vi "testing_delay_sweep_multifold_4ch.vi"() -> ()   [LabVIEW 2015, in "Tausand AB1000.lvlib"]
uses:
  <instrlib>/Tausand AB1000/Public/Controls/counters4ch.ctl
  <instrlib>/Tausand AB1000/Public/Controls/channelRing.ctl
  <instrlib>/Tausand AB1000/Public/Controls/configMultipleCoincRing.ctl
  <instrlib>/Tausand AB1000/Public/Controls/deviceTypeRing.ctl
  <instrlib>/Tausand AB1000/Tausand AB1000.lvlib
panel:
  out "device type":T1 items=["any"=0, "AB1002"=1002, "AB1004"=1004, "AB1502"=1502, "AB1504"=1504, "AB2002"=2002, "AB2004"=2004, "AB2502"=2502, "AB2504"=2504]
  out "multifold case":T2[](array[typedef])=[240, 224, 208, 176, 112] items=["ABC"=224, "ABD"=208, "ABE"=200, "ABF"=196, "ABG"=194, "ABH"=193, "ACD"=176, "ACE"=168, "ACF"=164, "ACG"=162, "ACH"=161, "ADE"=152, "ADF"=148, "ADG"=146, "ADH"=145, "AEF"=140, "AEG"=138, "AEH"=137, "AFG"=134, "AFH"=133, "AGH"=131, "BCD"=112, "BCE"=104, "BCF"=100, "BCG"=98, "BCH"=97, "BDE"=88, "BDF"=84, "BDG"=82, "BDH"=81, "BEF"=76, "BEG"=74, "BEH"=73, "BFG"=70, "BFH"=69, "BGH"=67, "CDE"=56, "CDF"=52, "CDG"=50, "CDH"=49, "CEF"=44, "CEG"=42, "CEH"=41, "CFG"=38, "CFH"=37, "CGH"=35, "DEF"=28, "DEG"=26, "DEH"=25, "DFG"=22, "DFH"=21, "DGH"=19, "EFG"=14, "EFH"=13, "EGH"=11, "FGH"=7, "ABCD"=240, "ABCE"=232, "ABCF"=228, "ABCG"=226, "ABCH"=225, "ABDE"=216, "ABDF"=212, "ABDG"=210, "ABDH"=209, "ABEF"=204, "ABEG"=202, "ABEH"=201, "ABFG"=198, "ABFH"=197, "ABGH"=195, "ACDE"=184, "ACDF"=180, "ACDG"=178, "ACDH"=177, "ACEF"=172, "ACEG"=170, "ACEH"=169, "ACFG"=166, "ACFH"=165, "ACGH"=163, "ADEF"=156, "ADEG"=154, "ADEH"=153, "ADFG"=150, "ADFH"=149, "ADGH"=147, "AEFG"=142, "AEFH"=141, "AEGH"=139, "AFGH"=135, "BCDE"=120, "BCDF"=116, "BCDG"=114, "BCDH"=113, "BCEF"=108, "BCEG"=106, "BCEH"=105, "BCFG"=102, "BCFH"=101, "BCGH"=99, "BDEF"=92, "BDEG"=90, "BDEH"=89, "BDFG"=86, "BDFH"=85, "BDGH"=83, "BEFG"=78, "BEFH"=77, "BEGH"=75, "BFGH"=71, "CDEF"=60, "CDEG"=58, "CDEH"=57, "CDFG"=54, "CDFH"=53, "CDGH"=51, "CEFG"=46, "CEFH"=45, "CEGH"=43, "CFGH"=39, "DEFG"=30, "DEFH"=29, "DEGH"=27, "DFGH"=23, "EFGH"=15]
  out "tausand data":u32[][](array[numeric])
  out "current multifold":T2=224 caption="Current multifold" items=["ABC"=224, "ABD"=208, "ABE"=200, "ABF"=196, "ABG"=194, "ABH"=193, "ACD"=176, "ACE"=168, "ACF"=164, "ACG"=162, "ACH"=161, "ADE"=152, "ADF"=148, "ADG"=146, "ADH"=145, "AEF"=140, "AEG"=138, "AEH"=137, "AFG"=134, "AFH"=133, "AGH"=131, "BCD"=112, "BCE"=104, "BCF"=100, "BCG"=98, "BCH"=97, "BDE"=88, "BDF"=84, "BDG"=82, "BDH"=81, "BEF"=76, "BEG"=74, "BEH"=73, "BFG"=70, "BFH"=69, "BGH"=67, "CDE"=56, "CDF"=52, "CDG"=50, "CDH"=49, "CEF"=44, "CEG"=42, "CEH"=41, "CFG"=38, "CFH"=37, "CGH"=35, "DEF"=28, "DEG"=26, "DEH"=25, "DFG"=22, "DFH"=21, "DGH"=19, "EFG"=14, "EFH"=13, "EGH"=11, "FGH"=7, "ABCD"=240, "ABCE"=232, "ABCF"=228, "ABCG"=226, "ABCH"=225, "ABDE"=216, "ABDF"=212, "ABDG"=210, "ABDH"=209, "ABEF"=204, "ABEG"=202, "ABEH"=201, "ABFG"=198, "ABFH"=197, "ABGH"=195, "ACDE"=184, "ACDF"=180, "ACDG"=178, "ACDH"=177, "ACEF"=172, "ACEG"=170, "ACEH"=169, "ACFG"=166, "ACFH"=165, "ACGH"=163, "ADEF"=156, "ADEG"=154, "ADEH"=153, "ADFG"=150, "ADFH"=149, "ADGH"=147, "AEFG"=142, "AEFH"=141, "AEGH"=139, "AFGH"=135, "BCDE"=120, "BCDF"=116, "BCDG"=114, "BCDH"=113, "BCEF"=108, "BCEG"=106, "BCEH"=105, "BCFG"=102, "BCFH"=101, "BCGH"=99, "BDEF"=92, "BDEG"=90, "BDEH"=89, "BDFG"=86, "BDFH"=85, "BDGH"=83, "BEFG"=78, "BEFH"=77, "BEGH"=75, "BFGH"=71, "CDEF"=60, "CDEG"=58, "CDEH"=57, "CDFG"=54, "CDFH"=53, "CDGH"=51, "CEFG"=46, "CEFH"=45, "CEGH"=43, "CFGH"=39, "DEFG"=30, "DEFH"=29, "DEGH"=27, "DFGH"=23, "EFGH"=15]
  in  "delayed channel":T3=1 items=["none", "A", "B", "C", "D", "E", "F", "G", "H"]
  in  "cw (ns)":u32=2
  out "i case":i32
  out "total cases":i32
  in  "Stop Button":bool
  out "coinc Chart":T4(graph)
  out "current values":T5
  in  "sampling (ms)":u32=1000
  out "i delay":i32
  out "delay array":u32[](array[numeric])
  in  "step delay":u32=2
  in  "max delay":u32=10
  in  "min delay":u32
  out "current delay (ns)":u32
  in  "VISA resource name":refnum<visa-resource-name>
  # "delayA"
  # "delayB"
  # "delayC"
  # "delayD"
  # "c.win."
  # "case"
  # "out of"
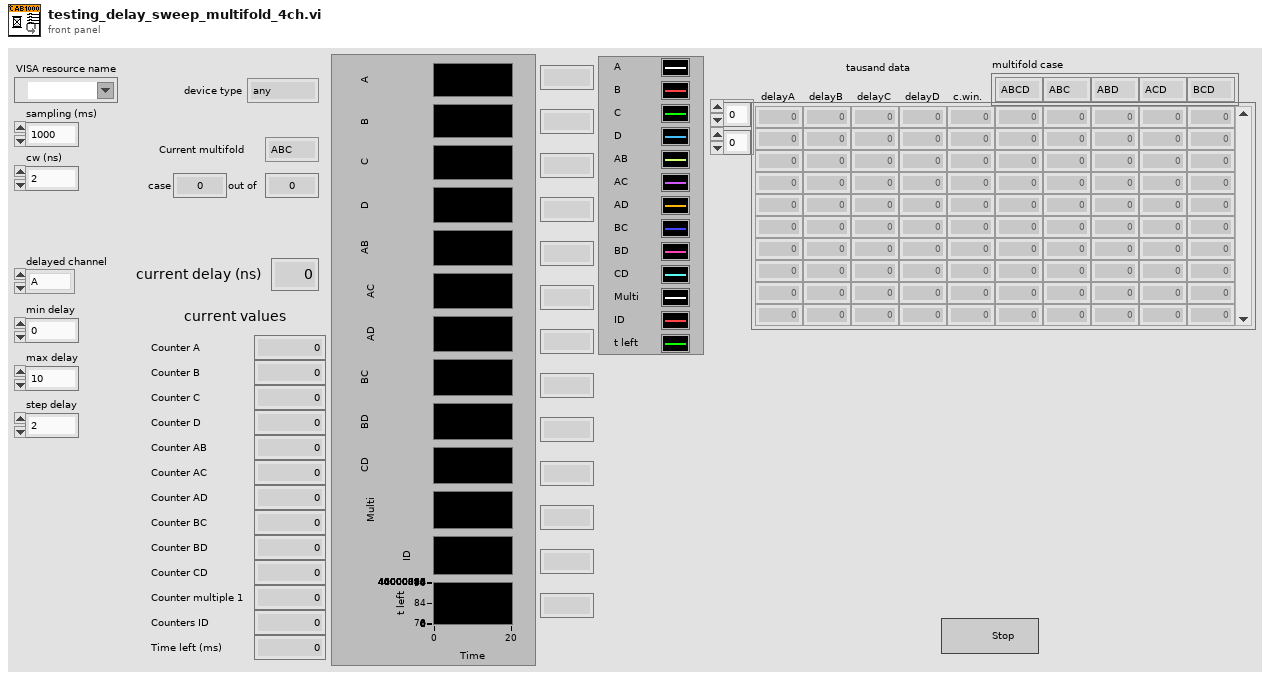
[diagram p1: front panel]
types:
  T1 = typedef "Tausand AB1000.lvlib/deviceTypeRing.ctl" = u16
  T2 = typedef "Tausand AB1000.lvlib/configMultipleCoincRing.ctl" = u16
  T3 = typedef "Tausand AB1000.lvlib/channelRing.ctl" = u8
  T4 = cluster{"counter_A":u32, "counter_B":u32, "counter_C":u32, "counter_D":u32, "counter_AB":u32, "counter_AC":u32, "counter_AD":u32, "counter_BC":u32, "counter_BD":u32, "counter_CD":u32, "counter_multiple_1":u32, "counters_ID":u32, "time_left":u32}
  T5 = typedef "Tausand AB1000.lvlib/counters4ch.ctl" = cluster{"counter_A":u32, "counter_B":u32, "counter_C":u32, "counter_D":u32, "counter_AB":u32, "counter_AC":u32, "counter_AD":u32, "counter_BC":u32, "counter_BD":u32, "counter_CD":u32, "counter_multiple_1":u32, "counters_ID":u32, "time_left":u32}
  T6 = typedef "Tausand AB1000.lvlib/settings4ch.ctl" = cluster{"sampling":u32, "coincidence_window":u32, "delay_A":u32, "delay_B":u32, "delay_C":u32, "delay_D":u32, "sleep_A":u32, "sleep_B":u32, "sleep_C":u32, "sleep_D":u32, "config_multiple_1":T2}
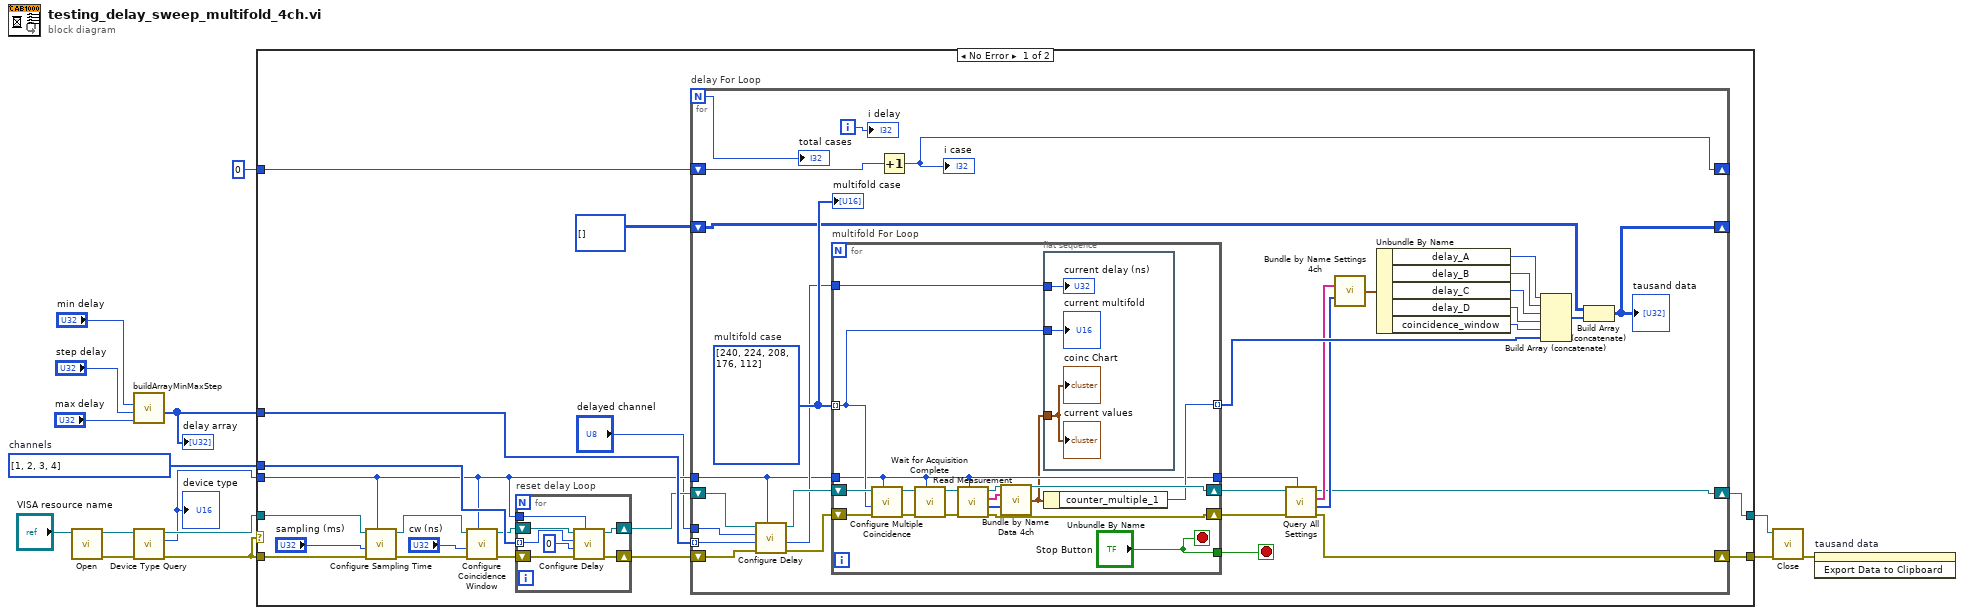
[diagram p0: block diagram]
diagram:
  w6 = T3[] [1, 2, 3, 4] items=["none", "A", "B", "C", "D", "E", "F", "G", "H"]  # channels
  n1 = call <instrlib>:"Open.vi"("VISA resource name"="VISA resource name") -> ("error out"=w11:errorcluster, "VISA resource name out"=w10:refnum<visa-resource-name>)  [unwired: 9 in]
  n2 = call <instrlib>:"buildArrayMinMaxStep.vi"("max (10)"="max delay", "step (1)"="step delay", "min (0)"="min delay") -> ("array"=w7:i32[])  [unwired: 8 in]
  "delay array" <- w7
  n3 = call <instrlib>:"Device Type Query.vi"("error in (no error)"=w11, "VISA Refnum in"=w10) -> ("error out"=w3:errorcluster, "device type"=w8:T1, "VISA Refnum out"=w9:refnum<visa-resource-name>)  [unwired: 7 in]
  "device type" <- w8
  n4 = case shown="No Error" w3 {
    tunnel: w3 -> [w28 w92]
    tunnel: w9 -> [w29 w91]
    tunnel: w8 -> [w27 _]
    tunnel: w7 -> [w33 _]
    tunnel: w6 -> [w30 _]
    tunnel: [w32 w91] -> w5
    tunnel: [w31 w92] -> w4
    tunnel: 0 ("i delay") -> [w23 _]
    frame No Error {
      n5 = call <instrlib>:"Configure Sampling Time.vi"("device type"=w27, "error in (no error)"=w28, "value (1000 ms)"="sampling (ms)", "VISA Refnum in"=w29) -> ("error out"=w25:errorcluster, "VISA Refnum out"=w24:refnum<visa-resource-name>)  [unwired: 5 in, 1 out]
      n6 = call <instrlib>:"Configure Coincidence Window.vi"("device type"=w27, "error in (no error)"=w25, "value ns (10ns)"="cw (ns)", "VISA Refnum in"=w24) -> ("error out"=w21:errorcluster, "VISA Refnum out"=w22:refnum<visa-resource-name>)  [unwired: 5 in, 1 out]
      n7 = for "reset delay Loop" {
        tunnel: w30 -> [w39] mode=indexing
        tunnel: w27 -> [w37]
        shift-right: [w35] -> w18
        shift-left: w21 -> [w36]
        shift-right: [w34] -> w19
        shift-left: w22 -> [w40]
        n8 = call <instrlib>:"Configure Delay.vi"("device type"=w37, "error in (no error)"=w36, "value (0 ns)"=u32 0, "channel"=w39, "VISA Refnum in"=w40) -> ("error out"=w35:errorcluster, "VISA Refnum out"=w34:refnum<visa-resource-name>)  [unwired: 4 in, 1 out]
      }
      n9 = for "delay For Loop" {
        N -> [w64]
        tunnel: w33 -> [w71] mode=indexing
        tunnel: w27 -> [w42]
        shift-right: [w45] -> w31
        shift-left: w18 -> [w69]
        shift-right: [w44] -> w32
        shift-left: w19 -> [w70]
        shift-right: [w66] -> _
        shift-left: w23 -> [w67]
        tunnel: "delayed channel" -> [w65]
        shift-right: [w57] -> _
        shift-left: u32[][] [] ("tausand data") -> [w59]
        i -> [w68]
        stop <- w43 stop-if-true
        w61 = T2[] [240, 224, 208, 176, 112] items=["ABC"=224, "ABD"=208, "ABE"=200, "ABF"=196, "ABG"=194, "ABH"=193, "ACD"=176, "ACE"=168, "ACF"=164, "ACG"=162, "ACH"=161, "ADE"=152, "ADF"=148, "ADG"=146, "ADH"=145, "AEF"=140, "AEG"=138, "AEH"=137, "AFG"=134, "AFH"=133, "AGH"=131, "BCD"=112, "BCE"=104, "BCF"=100, "BCG"=98, "BCH"=97, "BDE"=88, "BDF"=84, "BDG"=82, "BDH"=81, "BEF"=76, "BEG"=74, "BEH"=73, "BFG"=70, "BFH"=69, "BGH"=67, "CDE"=56, "CDF"=52, "CDG"=50, "CDH"=49, "CEF"=44, "CEG"=42, "CEH"=41, "CFG"=38, "CFH"=37, "CGH"=35, "DEF"=28, "DEG"=26, "DEH"=25, "DFG"=22, "DFH"=21, "DGH"=19, "EFG"=14, "EFH"=13, "EGH"=11, "FGH"=7, "ABCD"=240, "ABCE"=232, "ABCF"=228, "ABCG"=226, "ABCH"=225, "ABDE"=216, "ABDF"=212, "ABDG"=210, "ABDH"=209, "ABEF"=204, "ABEG"=202, "ABEH"=201, "ABFG"=198, "ABFH"=197, "ABGH"=195, "ACDE"=184, "ACDF"=180, "ACDG"=178, "ACDH"=177, "ACEF"=172, "ACEG"=170, "ACEH"=169, "ACFG"=166, "ACFH"=165, "ACGH"=163, "ADEF"=156, "ADEG"=154, "ADEH"=153, "ADFG"=150, "ADFH"=149, "ADGH"=147, "AEFG"=142, "AEFH"=141, "AEGH"=139, "AFGH"=135, "BCDE"=120, "BCDF"=116, "BCDG"=114, "BCDH"=113, "BCEF"=108, "BCEG"=106, "BCEH"=105, "BCFG"=102, "BCFH"=101, "BCGH"=99, "BDEF"=92, "BDEG"=90, "BDEH"=89, "BDFG"=86, "BDFH"=85, "BDGH"=83, "BEFG"=78, "BEFH"=77, "BEGH"=75, "BFGH"=71, "CDEF"=60, "CDEG"=58, "CDEH"=57, "CDFG"=54, "CDFH"=53, "CDGH"=51, "CEFG"=46, "CEFH"=45, "CEGH"=43, "CFGH"=39, "DEFG"=30, "DEFH"=29, "DEGH"=27, "DFGH"=23, "EFGH"=15]  # multifold case
        n10 = call <instrlib>:"Configure Delay.vi"("device type"=w42, "error in (no error)"=w69, "value (0 ns)"=w71, "channel"=w65, "VISA Refnum in"=w70) -> ("error out"=w63:errorcluster, "value ns out"=w56:u32, "VISA Refnum out"=w62:refnum<visa-resource-name>)  [unwired: 4 in]
        n11 = for "multifold For Loop" {
          tunnel: w56 -> [w78]
          tunnel: w42 -> [w73]
          shift-right: [w87] -> w55
          shift-left: w63 -> [w82]
          shift-right: [w86] -> w54
          shift-left: w62 -> [w80]
          tunnel: w61 -> [w77] mode=indexing
          tunnel: [w75] -> w60 mode=indexing
          tunnel: ["Stop Button"] -> w43
          tunnel: [w73] -> w41
          stop <- "Stop Button" stop-if-true
          n12 = call <instrlib>:"Configure Multiple Coincidence.vi"("device type"=w73, "error in (no error)"=w82, "Multiple coincidence configuration"=w77, "VISA Refnum in"=w80) -> ("error out"=w81:errorcluster, "VISA Refnum out"=w79:refnum<visa-resource-name>)  [unwired: 6 in]
          n13 = call <instrlib>:"Wait for Acquisition Complete.vi"("device type"=w73, "error in (no error)"=w81, "VISA resource name"=w79) -> ("error out"=w85:errorcluster, "VISA resource name out"=w84:refnum<visa-resource-name>)  [unwired: 7 in]
          n14 = call <instrlib>:"Read Measurement.vi"("device type"=w73, "error in (no error)"=w85, "VISA Refnum in"=w84) -> ("error out"=w87:errorcluster, "values"=w76:u32[], "labels"=w83:string[], "VISA Refnum out"=w86:refnum<visa-resource-name>)  [unwired: 3 in, 2 out]
          n15 = call <instrlib>:"Bundle by Name Data 4ch.vi"("names"=w83, "values"=w76) -> ("output cluster 4ch"=w72:T5)  [unwired: 13 in]
          n16 = flat-sequence {
            tunnel: w72 -> [w90]
            tunnel: w78 -> [w89]
            tunnel: w77 -> [w88]
            frame #0 {
              "current values" <- w90
              "coinc Chart" <- w90
              "current delay (ns)" <- w89
              "current multifold" <- w88
            }
          }
          n17 = Unbundle By Name(w72) -> ("counter_multiple_1"=w75:u32)
        }
        n18 = Increment(x=w67) -> (x+1=w66:i32)
        "i case" <- w66
        n19 = call <instrlib>:"Query All Settings.vi"("device type"=w41, "error in (no error)"=w55, "VISA Refnum in"=w54) -> ("error out"=w45:errorcluster, "values"=w52:u32[], "labels"=w53:string[], "VISA Refnum out"=w44:refnum<visa-resource-name>)  [unwired: 4 in, 1 out]
        n20 = call <instrlib>:"Bundle by Name Settings 4ch.vi"("names"=w53, "values"=w52) -> ("output cluster settings 4ch"=w51:T6)  [unwired: 13 in]
        n21 = Unbundle By Name(w51) -> ("delay_A"=w50:u32, "delay_B"=w49:u32, "delay_C"=w48:u32, "delay_D"=w47:u32, "coincidence_window"=w46:u32)
        n22 = Build Array (concatenate)(w50, w49, w48, w47, w46, w60) -> (w58:u32[])
        n23 = Build Array (concatenate)(w59, w58) -> (w57:u32[][])
        "tausand data" <- w57
        "i delay" <- w68
        "total cases" <- w64
        "multifold case" <- w61
      }
    }
    frame Error {
    }
  }
  n24 = call <instrlib>:"Close.vi"("error in (no error)"=w4, "VISA resource name"=w5) -> ("error out"=w1:errorcluster)  [unwired: 9 in]
  n25 = invoke on="tausand data" class="Arr (strict)" method="Export Data to Clipboard"(error in=w1) -> ()  [unwired: 2 in, 3 out]
